vi "Test App App Process Added Before Start Receives All Process Messages.vi"(8 "error in (no error)":errorcluster, 11 "Application Test In":refnum<class "Application Dev Test.lvclass">) -> (0 "error out":errorcluster, 3 "Application Test Out":refnum<class "Application Dev Test.lvclass">)   [LabVIEW 2020, in "Application Dev Test.lvclass"]
uses:
  Application Dev Test.lvclass
  C:/Program Files (x86)/National Instruments/LabVIEW 2020/vi.lib/Astemes/LUnit/Test Case.lvclass
  source/Framework Test Suite/Mock Process/Mock Process.lvclass
  C:/Git/astemes-triarc-framework/source/Framework/Process/Process.lvclass
  source/Framework/Process/Process.lvclass/Process.ctl
  source/Framework/Application/Application.lvclass/Application.ctl
  <vilib>/Astemes/LUnit/Test Case.lvclass/Test Case.ctl
  source/Framework/Application/Private/Add Process to Map.vi
  source/Framework/Application/Private/Throw Error If Process Already in App.vi
  source/Framework/Process/Protected/Messaging/Send Message.vi
  source/Framework/Process/Public/Lifecycle/Get Lifecycle State.vi
  source/Framework/Process/Protected/SubVIs/Set Context.vi
  source/Framework/Process/Private/SubVIs/Wait for finish.vi
  source/Framework/Process/Private/SubVIs/Set Lifecycle State.vi
  <vilib>/Astemes/LUnit/Palette/Fail.vi
  <vilib>/Astemes/LUnit/Palette/Pass.vi
  <vilib>/Astemes/LUnit/Set Assertion Type.vi
  source/Framework/Application/Public/Get Process.vi
  source/Framework/Process/Private/SubVIs/Handle Debug Data.vi
  <vilib>/Utility/error.llb/Clear Errors.vi
  source/Framework/Process/Public/Lifecycle/Leave Process Loop.vi
  <vilib>/Astemes/LUnit/Add test result.vi
  source/Framework/Application/Private/Retrieve Process from App.vi
  source/Framework/Application/Private/Parse Process Name.vi
  source/Framework/Application/Private/Get Process from Map.vi
  source/Framework/Logging/Log Debug.vi
  <vilib>/AdvancedString/1D String Array to Delimited String.vi
  <vilib>/Utility/High Resolution Relative Seconds.vi
  <vilib>/Astemes/LUnit/LUnit Record Assertion Result.vi
  source/Framework/Process/Protected/Messaging/Request Message.vi
  <vilib>/AdvancedString/Delimited String to 1D String Array.vi
  <vilib>/Astemes/LUnit/LUnit Aggregate Assertion Results.vi
  source/Framework/Process/Private/SubVIs/Enqueue Request Message.vi
  <vilib>/Astemes/LUnit/Method Result/LUnit Merge Status.vi
  <vilib>/Astemes/LUnit/LUnit Concatenate result strings.vi
  source/Framework/Application/Application.lvclass
  <vilib>/Utility/error.llb/Error Cluster From Error Code.vi
  source/Framework/Process/Public/Read Name.vi
  source/Framework/Process/Private/SubVIs/Wait for Response Message.vi
  source/Framework/Process/Process.lvclass
  <vilib>/Astemes/LUnit/Test Case.lvclass
panel:
  out "Messages":string[](array[string])
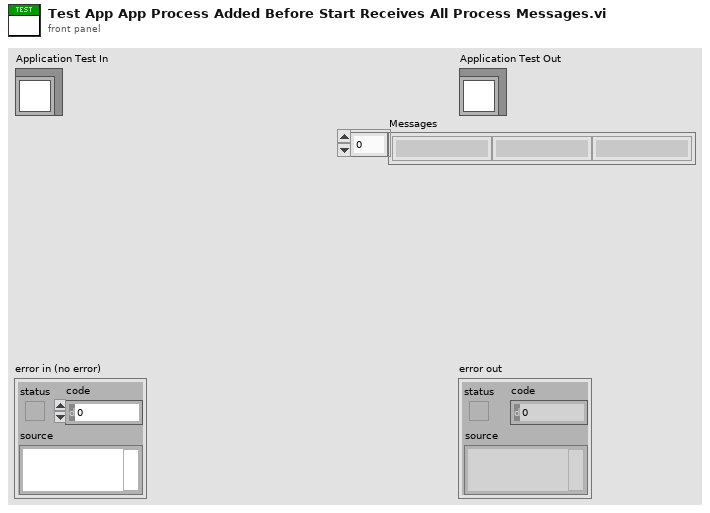
[diagram p1: front panel]
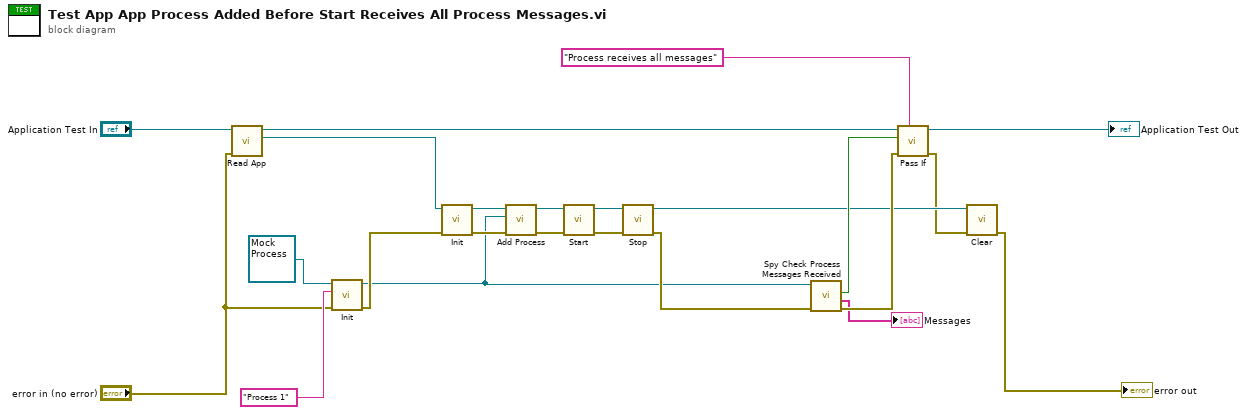
[diagram p0: block diagram]
diagram:
  n1 = call "Read App.vi"("error in (no error)"="error in (no error)", "Application Test In"="Application Test In") -> ("App out"=w16:refnum<class "Application.lvclass">, "Application Test Out"=w22:refnum<class "Application Dev Test.lvclass">)  [unwired: 7 in, 1 out]
  n2 = call-dynamic "Init.vi"("error in (no error)"="error in (no error)", "Name"="Process 1", "Mock Process In"=refnum<class "Mock Process.lvclass"> refnum ("Mock Classes.lvlib:Mock Process.lvclass")) -> ("error out"=w18:errorcluster, "Mock Process Out"=w17:refnum<class "Mock Process.lvclass">)  [unwired: 7 in]
  n3 = call-dynamic "Init.vi"("error in (no error)"=w18, "Process In"=w16) -> ("error out"=w20:errorcluster, "Process Out"=w21:refnum<class "Application.lvclass">)  [unwired: 8 in]
  n4 = call "Add Process.vi"("error in (no error)"=w20, "Process"=w17, "Application In"=w21) -> ("error out"=w11:errorcluster, "Application Out"=w14:refnum<class "Application.lvclass">)  [unwired: 7 in]
  n5 = call "Start.vi"("error in (no error)"=w11, "Process In"=w14) -> ("error out"=w12:errorcluster, "Process Out"=w13:refnum<class "Application.lvclass">)  [unwired: 7 in, 1 out]
  n6 = call "Stop.vi"("error in (no error)"=w12, "Process In"=w13) -> ("error out"=w19:errorcluster, "Process Out"=w3:refnum<class "Application.lvclass">)  [unwired: 7 in, 1 out]
  n7 = call "Spy Check Process Messages Received.vi"("error in (no error)"=w19, "Mock Process In"=w17) -> ("error out"=w9:errorcluster, "Messages"=→"Messages":string[], "Messages received?"=w8:bool)  [unwired: 6 in, 1 out]
  n8 = call <vilib>:"Pass If.vi"("Description"="Process receives all messages", "error in (no error)"=w9, "Pass?"=w8, "LUnit Test Case In"=w22) -> ("error out"=w2:errorcluster, "LUnit Test Case Out"=→"Application Test Out":refnum<class "Application Dev Test.lvclass">)  [unwired: 6 in]
  n9 = call-dynamic "Clear.vi"("error in (no error)"=w2, "Application In"=w3) -> ("error out"=→"error out":errorcluster)  [unwired: 9 in]
